vi "Refresh Auth.vi"(7 "Required Scope(s)":string[](array[string]), 8 "error in (no error)":errorcluster, 9 "Timeout S (60)":dbl=60.0, 10 "Authorization in":refnum<class "Authorization.lvclass">, 11 "OAuth2 in":refnum<class "OAuth2.lvclass">) -> (0 "error out":errorcluster, 1 "Async Authentication":refnum<class "Async Authorization.lvclass">, 3 "OAuth2 out":refnum<class "OAuth2.lvclass">)   [LabVIEW 2020, in "OAuth2.lvlib" / "OAuth2.lvclass"]
doc: "Attempts to refresh the authorization token based on an existing valid but expired authorization. This requires no interaction from a user as long as OAuth is configured correctly and the existing authorization has a valid refresh token.\n\nIf the user should be prompted for authorization if their credentials are no longer valid, use <b>Do Async Auth.vi</b> instead."
uses:
  OAuth2.lvclass
  Authorization/Authorization.lvclass
  Async Authorization/Async Authorization.lvclass
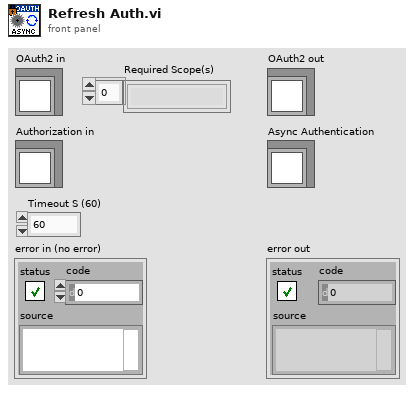
[diagram p1: front panel]
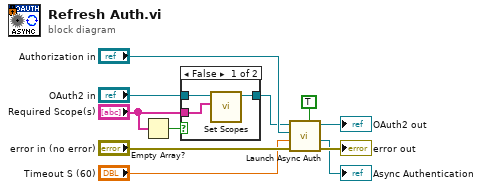
[diagram p0: block diagram]
diagram:
  n1 = Empty Array?(array="Required Scope(s)") -> (empty?=w4:bool)
  n2 = case shown="False" w4 {
    tunnel: "Required Scope(s)" -> [w12 _]
    tunnel: "OAuth2 in" -> [w14 w15]
    tunnel: [w13 w15] -> w1
    frame False {
      n3 = call "Set Scopes.vi"("Scopes"=w12, "OAuth2 in"=w14) -> ("OAuth2 out"=w13:refnum<class "OAuth2.lvclass">)  [unwired: 8 in, 1 out]
    }
    frame True {
    }
  }
  n4 = call "Launch Async Auth.vi"("Refresh Only?"=TRUE, "error in (no error)"="error in (no error)", "Timeout S (60)"="Timeout S (60)", "Authorization in"="Authorization in", "OAuth2 in"=w1) -> ("error out"=→"error out":errorcluster, "Async Authentication"=→"Async Authentication":refnum<class "Async Authorization.lvclass">, "OAuth2 out"=→"OAuth2 out":refnum<class "OAuth2.lvclass">)  [unwired: 4 in]
